vi "changeTarget.vi"(8 "error in (no error)":errorcluster, 9 "targetNumber":i16, 10 "interface object in":refnum<k20>, 11 "MotorController in":refnum<class "MotorController.lvclass">) -> (0 "error out":errorcluster, 1 "changeTargetRes":u32, 2 "interface object out":refnum<k20>, 3 "MotorController out":refnum<class "MotorController.lvclass">)   [LabVIEW 2018, in "MotorController.lvclass"]
uses:
  MotorController.lvclass
  MotorController.lvclass/MotorController.ctl
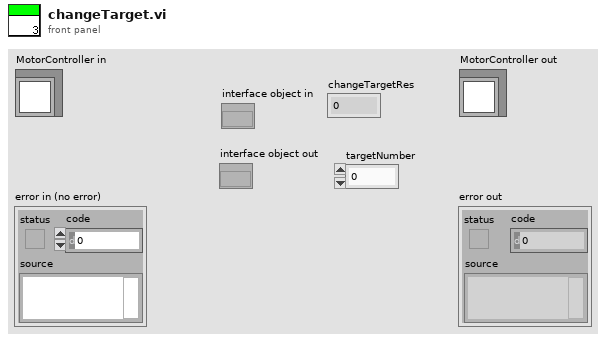
[diagram p1: front panel]
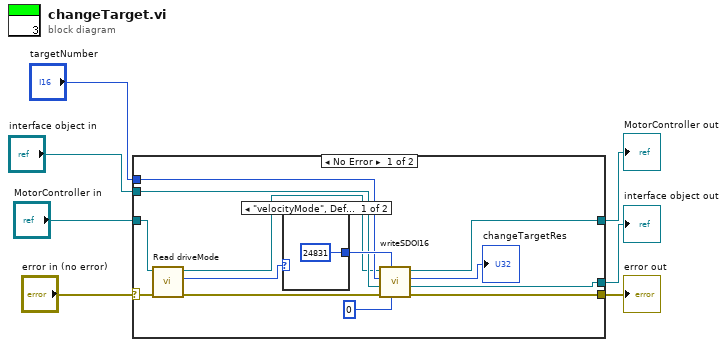
[diagram p0: block diagram]
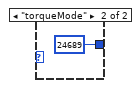
[diagram p2: hidden frame]
diagram:
  n1 = case shown="No Error" "error in (no error)" {
    selector: "error in (no error)" -> [w10 w25]
    tunnel: [w15 w25] -> w6
    tunnel: [w13 w24] -> w4
    tunnel: "MotorController in" -> [w12 w24]
    tunnel: "targetNumber" -> [w18 _]
    tunnel: "interface object in" -> [w17 w23]
    tunnel: [w16 w23] -> w1
    frame No Error {
      n2 = call "Read driveMode.vi"("error in (no error)"=w10, "MotorController in"=w12) -> ("error out"=w9:errorcluster, "driveMode"=w8:enum16{"velocityMode", "torqueMode", ""}, "MotorController out"=w11:refnum<class "MotorController.lvclass">)  [unwired: 7 in]
      n3 = case shown="\"velocityMode\", Default" w8 {
        tunnel: [u16 24831 ("object index") u16 24689 ("object index")] -> w20
        frame "velocityMode", Default {
        }
        frame "torqueMode" {
        }
      }
      n4 = call "writeSDOI16.vi"("object sub-index (0)"=u8 0, "object index"=w20, "error in (no error)"=w9, "interface object in"=w17, "inputNumber"=w18, "MotorController in"=w11) -> ("error out"=w15:errorcluster, "interface object out"=w16:refnum<k20>, "completion code"=→"changeTargetRes":u32, "MotorController out"=w13:refnum<class "MotorController.lvclass">)  [unwired: 2 in]
    }
    frame Error {
    }
  }
  "error out" <- w6
  "MotorController out" <- w4
  "interface object out" <- w1
